vi "Connect AOD.vi"(8 "error in (no error)":errorcluster, 10 "AOD Status In":T2={"AOD State"=enum."Idle", "daq task"="", "AOD Configuration"={"Physical Channel"="Dev1/ao0:1", "Maximum Value"=10.0, "Minimum Value"=1.0, "Update Rate"=192000.0}} {"AOD Configuration"."Update Rate" format="%0.2f"; "AOD Configuration"."Minimum Value" format="%0.2f"; "AOD Configuration"."Maximum Value" format="%0.2f"}, 11 "AOD Configuration":T1 {"Update Rate" format="%0.2f"; "Minimum Value" format="%0.2f"; "Maximum Value" format="%0.2f"}) -> (0 "error out":errorcluster, 3 "AOD Status Out":T2={"AOD State"=enum."Idle", "daq task"="", "AOD Configuration"={"Physical Channel"="Dev1/ao0:1", "Maximum Value"=10.0, "Minimum Value"=1.0, "Update Rate"=192000.0}} {"AOD Configuration"."Update Rate" format="%0.2f"; "AOD Configuration"."Minimum Value" format="%0.2f"; "AOD Configuration"."Maximum Value" format="%0.2f"})   [LabVIEW 2015, in "AOD.lvlib"]
uses:
  AOD.lvlib
  AOD State.ctl
  AOD Loop State.ctl
  AOD Configuration.ctl
  <vilib>/DAQmx/create/channels.llb/DAQmx Create Channel (AO-Voltage-Basic).vi
  <vilib>/DAQmx/configure/timing.llb/DAQmx Timing (Sample Clock).vi
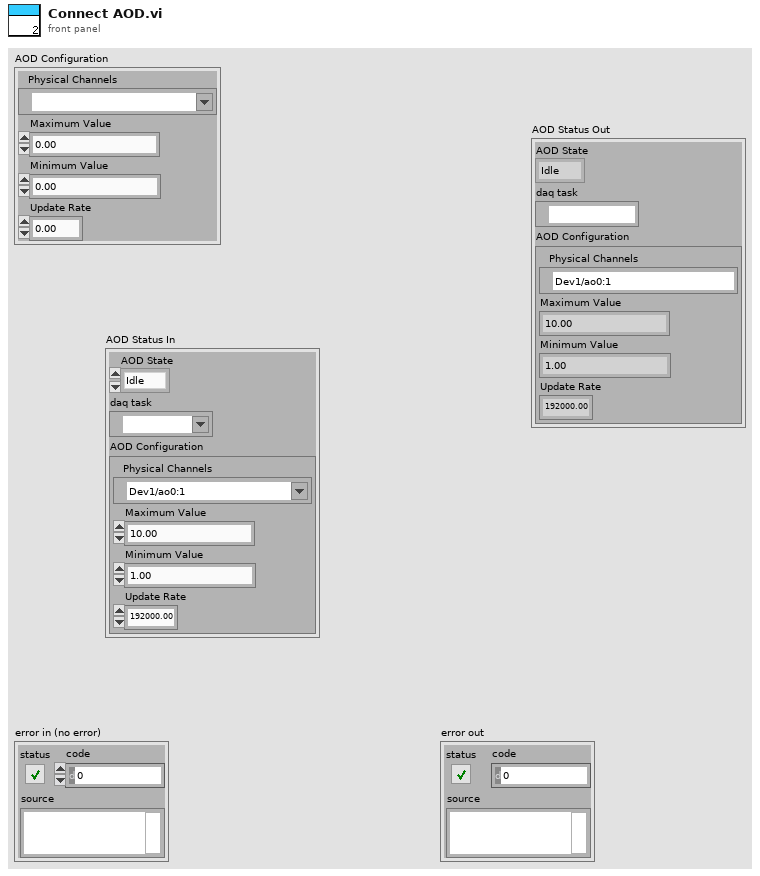
[diagram p1: front panel]
types:
  T1 = typedef "AOD.lvlib/AOD Configuration.ctl" = cluster{"Physical Channel":tag, "Maximum Value":dbl, "Minimum Value":dbl, "Update Rate":dbl}
  T2 = typedef "AOD.lvlib/AOD State.ctl" = cluster{"AOD State":T3, "daq task":refnum<k21>, "AOD Configuration":T1}
  T3 = typedef "AOD.lvlib/AOD Loop State.ctl" = enum16{"Idle", "Connected"}
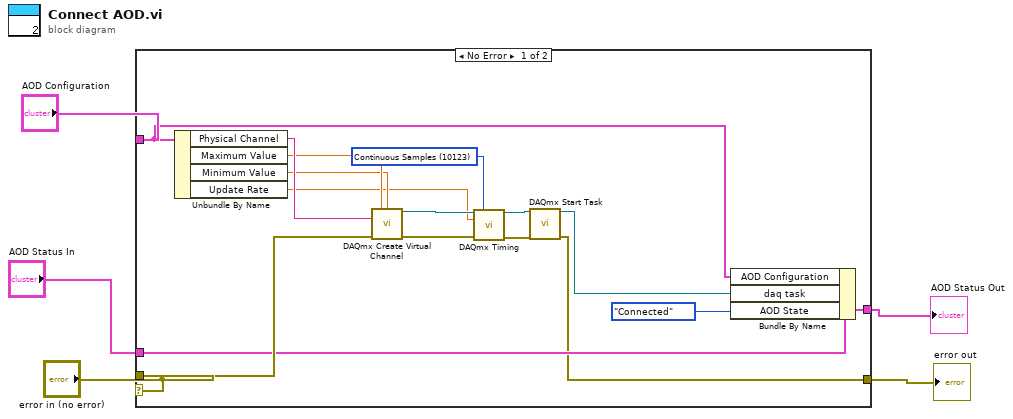
[diagram p0: block diagram]
diagram:
  n1 = case shown="No Error" "error in (no error)" {
    tunnel: [w6 w22] -> w5
    tunnel: "error in (no error)" -> [w21 w22]
    tunnel: "AOD Status In" -> [w18 w23]
    tunnel: [w17 w23] -> w3
    tunnel: "AOD Configuration" -> [w10 _]
    frame No Error {
      w11 = 10123 items=["Finite Samples"=10178, "Continuous Samples"=10123, "Hardware Timed Single Point"=12522] ("sample mode")
      n2 = Unbundle By Name(w10) -> ("Physical Channel"=w16:tag, "Maximum Value"=w14:dbl, "Minimum Value"=w13:dbl, "Update Rate"=w12:dbl)
      n3 = call-poly <vilib>:"DAQmx Create Virtual Channel.vi"("maximum value"=w14, "minimum value"=w13, "physical channels"=w16, "error in"=w21) -> ("task out"=w20:refnum<k21>, "error out"=w15:errorcluster)  [unwired: 10 in]
      n4 = call-poly <vilib>:"DAQmx Timing.vi"("task/channels in"=w20, "sample mode"=w11, "rate"=w12, "error in"=w15) -> ("task out"=w9:refnum<k21>, "error out"=w7:errorcluster)  [unwired: 10 in]
      n5 = call <vilib>:"DAQmx Start Task.vi"("task/channels in"=w9, "error in"=w7) -> ("task out"=w8:refnum<k21>, "error out"=w6:errorcluster)  [unwired: 12 in]
      n6 = Bundle By Name(cluster=w18, "AOD Configuration"=w10, "daq task"=w8, "AOD State"=AOD_Loop_State."Connected") -> (w17:T2)
    }
    frame Error {
    }
  }
  "error out" <- w5
  "AOD Status Out" <- w3
